vi "cam0config-20GC.vi"(8 "error_in":errorcluster caption="错误输入（无错误）", 10 "Attribute Information Array":T3(array[cluster]), 11 "Session in":T1 caption="Session Out") -> (0 "error_out":errorcluster caption="错误输出", 3 "Session_out":T1)   [LabVIEW 2015]
uses:
  <vilib>/vision/driver/IMAQdx.llb/IMAQdx Attribute Type.ctl
  <vilib>/userdefined/High Color/IMAQdx.ctl
  <resource>/objmgr/imaqdx.rc
  <vilib>/vision/driver/NI_Vision_Acquisition_Software.lvlib
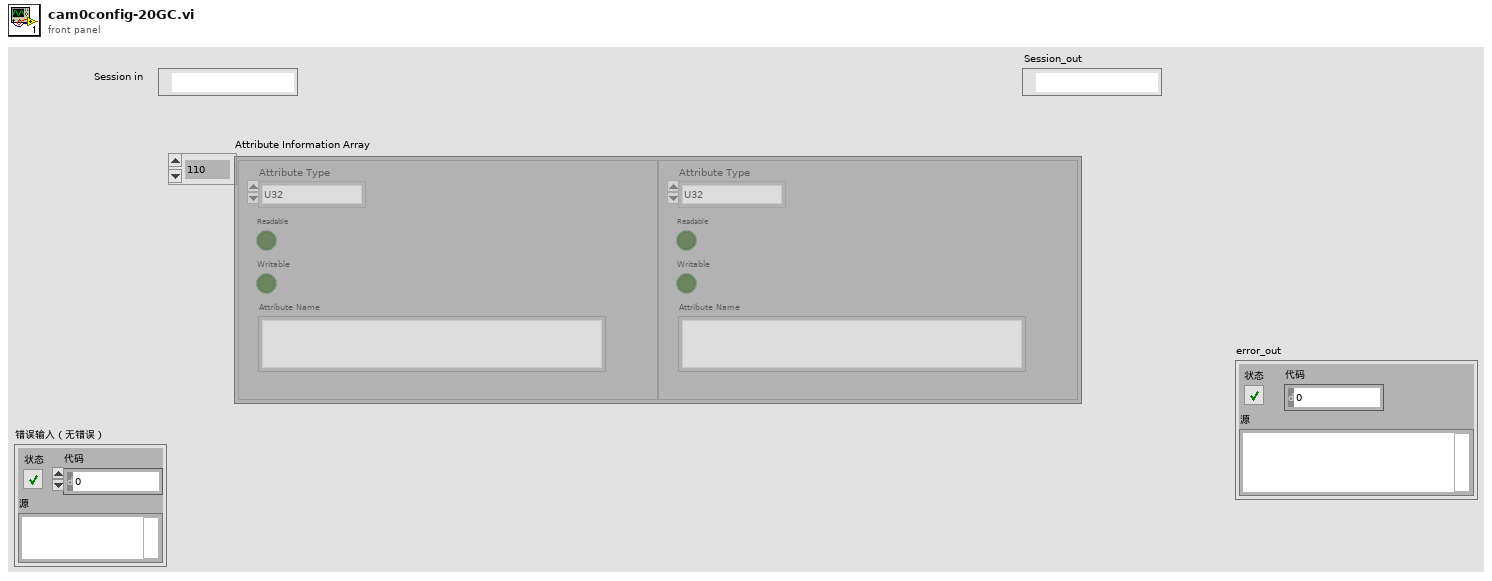
[diagram p1: front panel]
types:
  T1 = typedef "IMAQdx.ctl" = refnum<k21>
  T2 = typedef "NI_Vision_Acquisition_Software.lvlib/IMAQdx Attribute Type.ctl" = enum32{"U32", "I64", "DBL", "String", "Enum", "Bool", "Command"}
  T3 = cluster{"Attribute Type":T2, "Readable":bool, "Writable":bool, "Attribute Name":string}[]
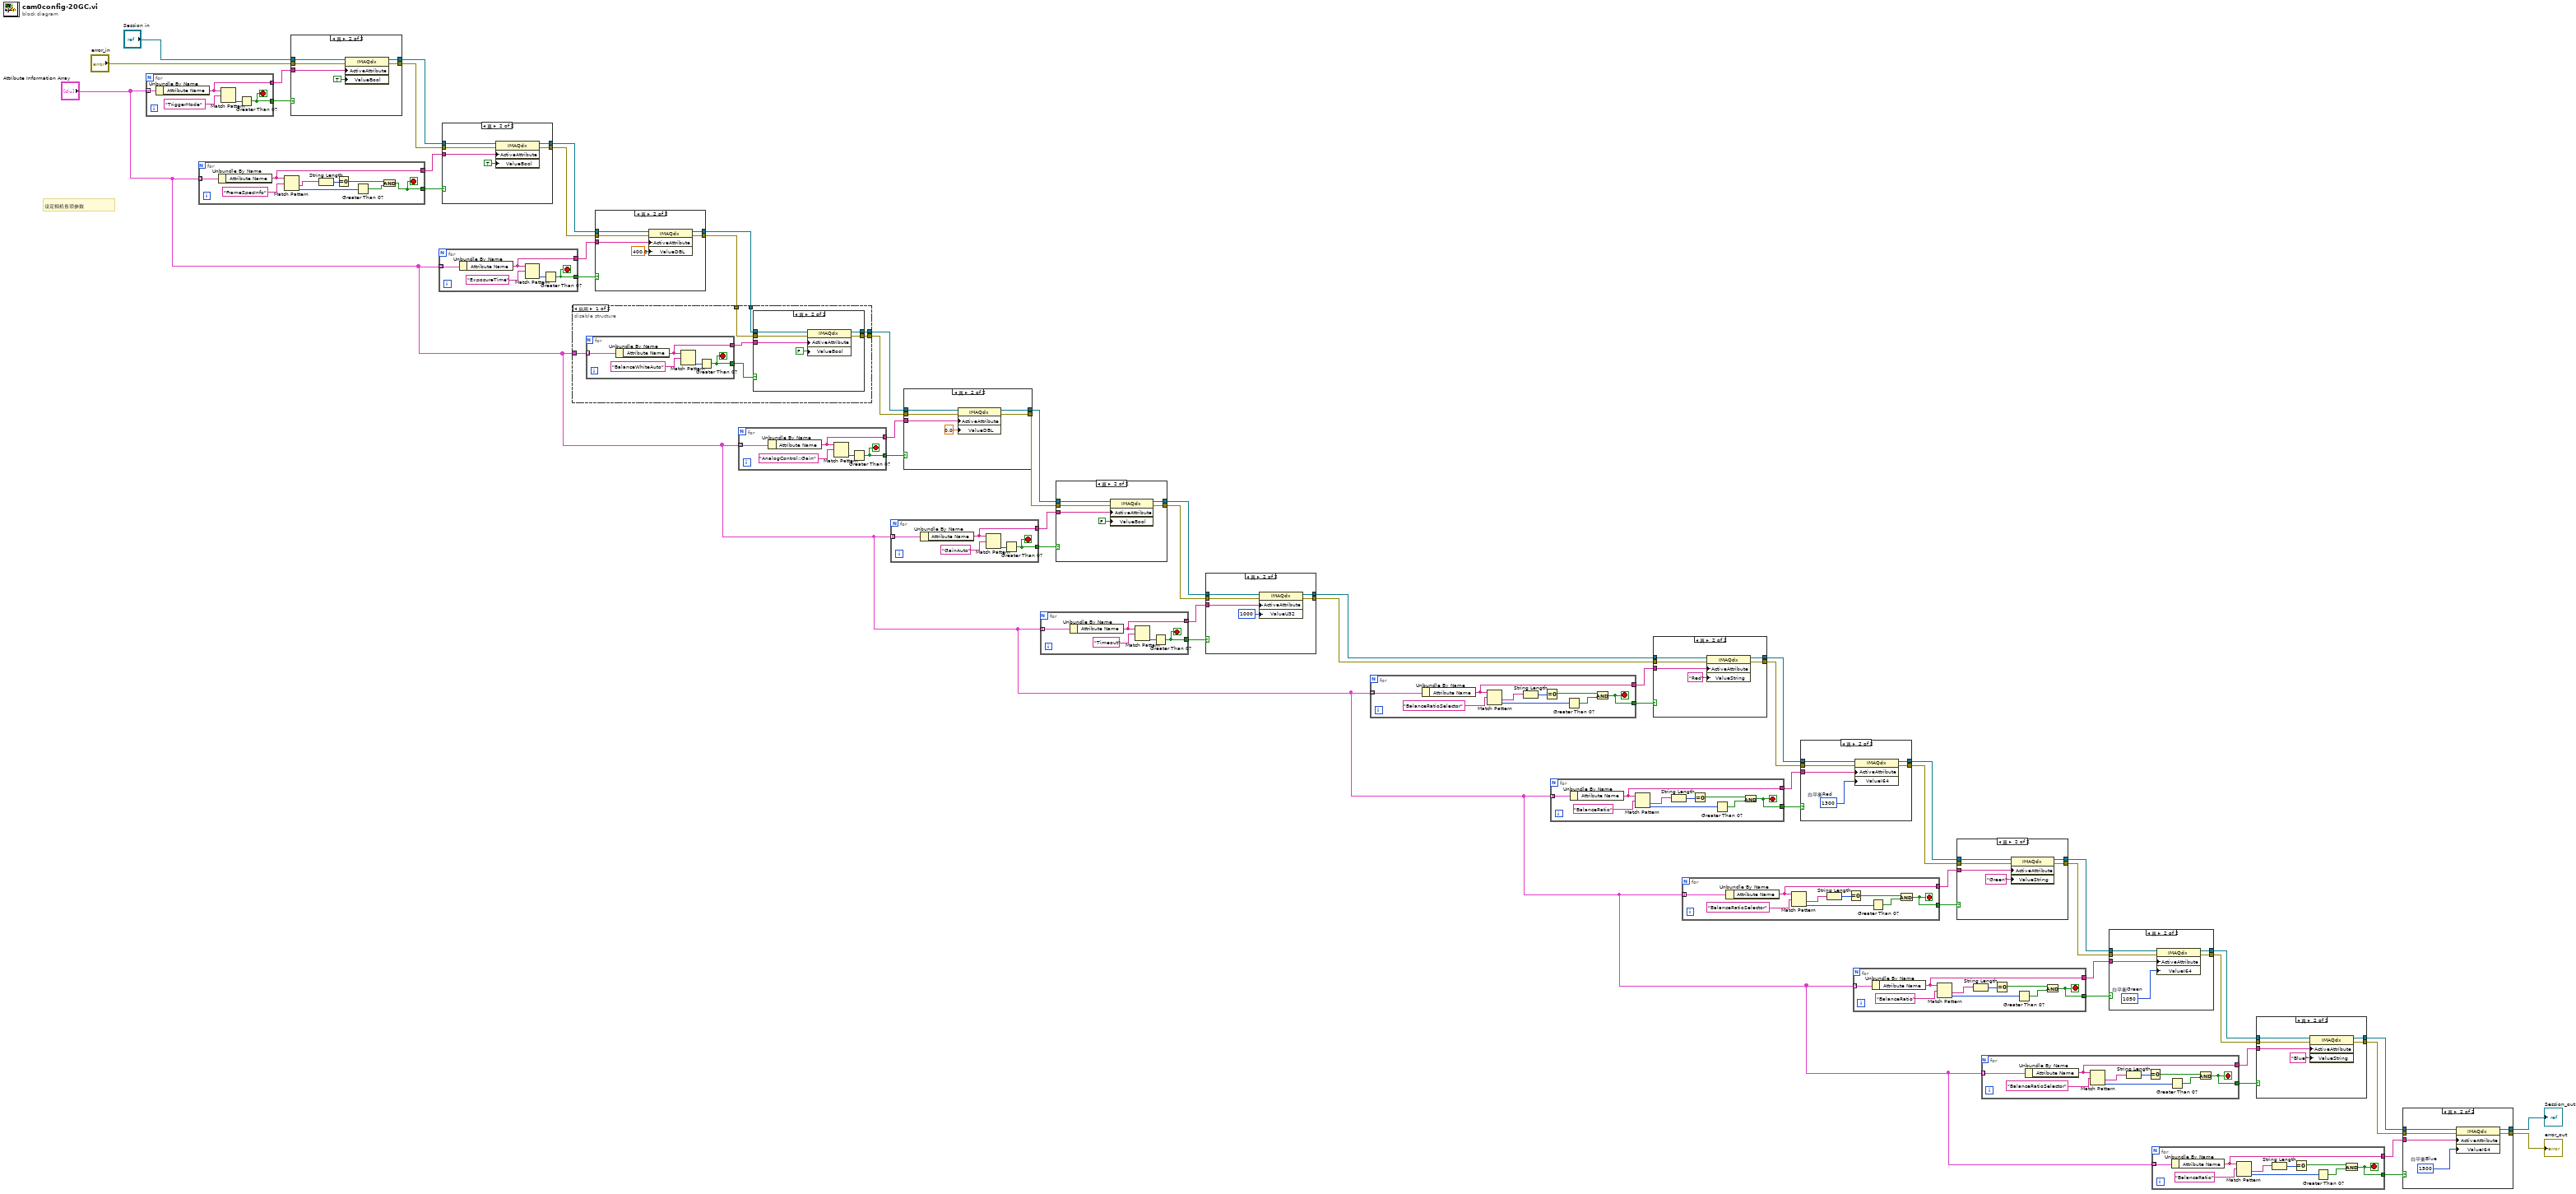
[diagram p0: block diagram]
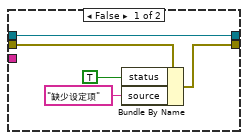
[diagram p2: hidden frame]
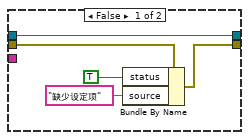
[diagram p3: hidden frame]
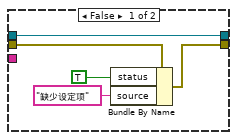
[diagram p4: hidden frame]
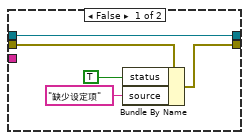
[diagram p5: hidden frame]
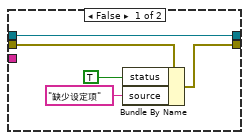
[diagram p6: hidden frame]
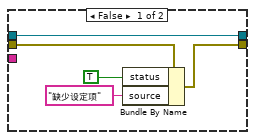
[diagram p7: hidden frame]
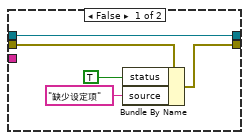
[diagram p8: hidden frame]
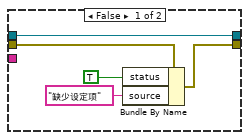
[diagram p10: hidden frame]
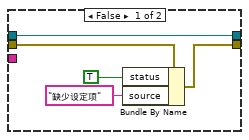
[diagram p11: hidden frame]
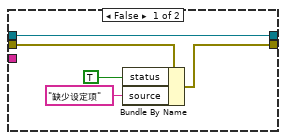
[diagram p12: hidden frame]
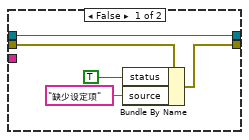
[diagram p13: hidden frame]
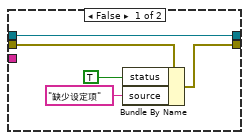
[diagram p14: hidden frame]
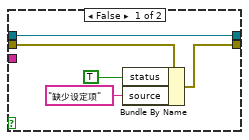
[diagram p15: hidden frame]
diagram:
  # "设定相机各项参数"
  n1 = for {
    tunnel: "Attribute Information Array" -> [w57] mode=indexing
    tunnel: [w55] -> w53
    tunnel: [w54] -> w52
    stop <- w55 stop-if-true
    n2 = Unbundle By Name(w57) -> ("Attribute Name"=w54:string)
    n3 = Match Pattern(string=w54, regular expression="TriggerMode" ("输入字符串")) -> (offset past match=w56:i32)  [unwired: 1 in, 3 out]
    n4 = Greater Than 0?(x=w56) -> (x > 0?=w55:bool)
  }
  n5 = for {
    tunnel: "Attribute Information Array" -> [w66] mode=indexing
    tunnel: [w60] -> w50
    tunnel: [w64] -> w51
    stop <- w60 stop-if-true
    n6 = Unbundle By Name(w66) -> ("Attribute Name"=w64:string)
    n7 = Match Pattern(string=w64, regular expression="FrameSpecInfo" ("输入字符串")) -> (after substring=w63:string, offset past match=w65:i32)  [unwired: 1 in, 2 out]
    n8 = String Length(string=w63) -> (length=w62:i32)
    n9 = Equal To 0?(x=w62) -> (x = 0?=w59:bool)
    n10 = Greater Than 0?(x=w65) -> (x > 0?=w61:bool)
    n11 = And(x=w59, y=w61) -> (x .and. y?=w60:bool)
  }
  n12 = case shown="真" w53 {
    tunnel: "Session in" -> [w72 w78]
    tunnel: w52 -> [_ w77]
    tunnel: [w72 w75] -> w49
    tunnel: "error_in" -> [w71 w74]
    tunnel: [w70 w73] -> w48
    frame False {
      n13 = Bundle By Name(cluster=w71, "status"=TRUE, "source"="缺少设定项") -> (w70:errorcluster)
    }
    frame True {
      n14 = property class="IMAQdx"(reference=w78, error in=w74, "ActiveAttribute"=w77, "ValueBool"=TRUE) -> (reference out=w75:T1, error out=w73:errorcluster)
    }
  }
  n15 = for {
    tunnel: "Attribute Information Array" -> [w82] mode=indexing
    tunnel: [w80] -> w47
    tunnel: [w79] -> w46
    stop <- w80 stop-if-true
    n16 = Unbundle By Name(w82) -> ("Attribute Name"=w79:string)
    n17 = Match Pattern(string=w79, regular expression="ExposureTime" ("输入字符串")) -> (offset past match=w81:i32)  [unwired: 1 in, 3 out]
    n18 = Greater Than 0?(x=w81) -> (x > 0?=w80:bool)
  }
  n19 = case shown="真" w50 {
    tunnel: w49 -> [w88 w94]
    tunnel: w51 -> [_ w93]
    tunnel: [w88 w91] -> w45
    tunnel: w48 -> [w87 w90]
    tunnel: [w86 w89] -> w44
    frame False {
      n20 = Bundle By Name(cluster=w87, "status"=TRUE, "source"="缺少设定项") -> (w86:errorcluster)
    }
    frame True {
      n21 = property class="IMAQdx"(reference=w94, error in=w90, "ActiveAttribute"=w93, "ValueBool"=TRUE) -> (reference out=w91:T1, error out=w89:errorcluster)
    }
  }
  n22 = case shown="真" w47 {
    tunnel: w45 -> [w99 w105]
    tunnel: w46 -> [_ w104]
    tunnel: [w99 w103] -> w43
    tunnel: w44 -> [w98 w102]
    tunnel: [w97 w101] -> w42
    frame False {
      n23 = Bundle By Name(cluster=w98, "status"=TRUE, "source"="缺少设定项") -> (w97:errorcluster)
    }
    frame True {
      n24 = property class="IMAQdx"(reference=w105, error in=w102, "ActiveAttribute"=w104, "ValueDBL"=400.0) -> (reference out=w103:T1, error out=w101:errorcluster)
    }
  }
  n25 = disable-structure shown="启用" {
    disable-tunnel: w43 -> [w110 w129]
    disable-tunnel: w42 -> [w109 w130]
    disable-tunnel: [w108 w129] -> w37
    disable-tunnel: [w107 w130] -> w36
    disable-tunnel: "Attribute Information Array" -> [w106 _]
    frame Enabled {
      n26 = for {
        tunnel: w106 -> [w127] mode=indexing
        tunnel: [w125] -> w111
        tunnel: [w124] -> w112
        stop <- w125 stop-if-true
        n27 = Unbundle By Name(w127) -> ("Attribute Name"=w124:string)
        n28 = Match Pattern(string=w124, regular expression="BalanceWhiteAuto" ("输入字符串")) -> (offset past match=w126:i32)  [unwired: 1 in, 3 out]
        n29 = Greater Than 0?(x=w126) -> (x > 0?=w125:bool)
      }
      n30 = case shown="真" w111 {
        tunnel: w110 -> [w117 w123]
        tunnel: w112 -> [_ w122]
        tunnel: [w117 w121] -> w108
        tunnel: w109 -> [w116 w120]
        tunnel: [w115 w119] -> w107
        frame False {
          n31 = Bundle By Name(cluster=w116, "status"=TRUE, "source"="缺少设定项") -> (w115:errorcluster)
        }
        frame True {
          n32 = property class="IMAQdx"(reference=w123, error in=w120, "ActiveAttribute"=w122, "ValueBool"=FALSE) -> (reference out=w121:T1, error out=w119:errorcluster)
        }
      }
    }
    frame Disabled {
    }
  }
  n33 = for {
    tunnel: "Attribute Information Array" -> [w134] mode=indexing
    tunnel: [w132] -> w41
    tunnel: [w131] -> w40
    stop <- w132 stop-if-true
    n34 = Unbundle By Name(w134) -> ("Attribute Name"=w131:string)
    n35 = Match Pattern(string=w131, regular expression="AnalogControl::Gain" ("输入字符串")) -> (offset past match=w133:i32)  [unwired: 1 in, 3 out]
    n36 = Greater Than 0?(x=w133) -> (x > 0?=w132:bool)
  }
  n37 = for {
    tunnel: "Attribute Information Array" -> [w139] mode=indexing
    tunnel: [w137] -> w38
    tunnel: [w136] -> w39
    stop <- w137 stop-if-true
    n38 = Unbundle By Name(w139) -> ("Attribute Name"=w136:string)
    n39 = Match Pattern(string=w136, regular expression="GainAuto" ("输入字符串")) -> (offset past match=w138:i32)  [unwired: 1 in, 3 out]
    n40 = Greater Than 0?(x=w138) -> (x > 0?=w137:bool)
  }
  n41 = case shown="真" w41 {
    tunnel: w37 -> [w145 w151]
    tunnel: w40 -> [_ w150]
    tunnel: [w145 w149] -> w35
    tunnel: w36 -> [w144 w148]
    tunnel: [w143 w147] -> w34
    frame False {
      n42 = Bundle By Name(cluster=w144, "status"=TRUE, "source"="缺少设定项") -> (w143:errorcluster)
    }
    frame True {
      n43 = property class="IMAQdx"(reference=w151, error in=w148, "ActiveAttribute"=w150, "ValueDBL"=0.0) -> (reference out=w149:T1, error out=w147:errorcluster)
    }
  }
  n44 = for {
    tunnel: "Attribute Information Array" -> [w155] mode=indexing
    tunnel: [w153] -> w31
    tunnel: [w152] -> w30
    stop <- w153 stop-if-true
    n45 = Unbundle By Name(w155) -> ("Attribute Name"=w152:string)
    n46 = Match Pattern(string=w152, regular expression="Timeout" ("输入字符串")) -> (offset past match=w154:i32)  [unwired: 1 in, 3 out]
    n47 = Greater Than 0?(x=w154) -> (x > 0?=w153:bool)
  }
  n48 = case shown="真" w38 {
    tunnel: w35 -> [w161 w167]
    tunnel: w39 -> [_ w166]
    tunnel: [w161 w165] -> w29
    tunnel: w34 -> [w160 w164]
    tunnel: [w159 w163] -> w28
    frame False {
      n49 = Bundle By Name(cluster=w160, "status"=TRUE, "source"="缺少设定项") -> (w159:errorcluster)
    }
    frame True {
      n50 = property class="IMAQdx"(reference=w167, error in=w164, "ActiveAttribute"=w166, "ValueBool"=FALSE) -> (reference out=w165:T1, error out=w163:errorcluster)
    }
  }
  n51 = case shown="真" w31 {
    tunnel: w29 -> [w172 w178]
    tunnel: w30 -> [_ w177]
    tunnel: [w172 w176] -> w3
    tunnel: w28 -> [w171 w175]
    tunnel: [w170 w174] -> w2
    frame False {
      n52 = Bundle By Name(cluster=w171, "status"=TRUE, "source"="缺少设定项") -> (w170:errorcluster)
    }
    frame True {
      n53 = property class="IMAQdx"(reference=w178, error in=w175, "ActiveAttribute"=w177, "ValueU32"=u32 1000) -> (reference out=w176:T1, error out=w174:errorcluster)
    }
  }
  n54 = for {
    tunnel: "Attribute Information Array" -> [w187] mode=indexing
    tunnel: [w180] -> w26
    tunnel: [w185] -> w27
    stop <- w180 stop-if-true
    n55 = Unbundle By Name(w187) -> ("Attribute Name"=w185:string)
    n56 = Match Pattern(string=w185, regular expression="BalanceRatioSelector" ("输入字符串")) -> (after substring=w183:string, offset past match=w186:i32)  [unwired: 1 in, 2 out]
    n57 = String Length(string=w183) -> (length=w184:i32)
    n58 = Equal To 0?(x=w184) -> (x = 0?=w182:bool)
    n59 = Greater Than 0?(x=w186) -> (x > 0?=w181:bool)
    n60 = And(x=w182, y=w181) -> (x .and. y?=w180:bool)
  }
  n61 = for {
    tunnel: "Attribute Information Array" -> [w196] mode=indexing
    tunnel: [w189] -> w25
    tunnel: [w194] -> w24
    stop <- w189 stop-if-true
    n62 = Unbundle By Name(w196) -> ("Attribute Name"=w194:string)
    n63 = Match Pattern(string=w194, regular expression="BalanceRatio" ("输入字符串")) -> (after substring=w192:string, offset past match=w195:i32)  [unwired: 1 in, 2 out]
    n64 = String Length(string=w192) -> (length=w193:i32)
    n65 = Equal To 0?(x=w193) -> (x = 0?=w191:bool)
    n66 = Greater Than 0?(x=w195) -> (x > 0?=w190:bool)
    n67 = And(x=w191, y=w190) -> (x .and. y?=w189:bool)
  }
  n68 = case shown="真" w26 {
    tunnel: w3 -> [w201 w207]
    tunnel: w27 -> [_ w206]
    tunnel: [w201 w205] -> w20
    tunnel: w2 -> [w200 w204]
    tunnel: [w199 w203] -> w21
    frame False {
      n69 = Bundle By Name(cluster=w200, "status"=TRUE, "source"="缺少设定项") -> (w199:errorcluster)
    }
    frame True {
      n70 = property class="IMAQdx"(reference=w207, error in=w204, "ActiveAttribute"=w206, "ValueString"="Red") -> (reference out=w205:T1, error out=w203:errorcluster)
    }
  }
  n71 = for {
    tunnel: "Attribute Information Array" -> [w216] mode=indexing
    tunnel: [w209] -> w22
    tunnel: [w214] -> w23
    stop <- w209 stop-if-true
    n72 = Unbundle By Name(w216) -> ("Attribute Name"=w214:string)
    n73 = Match Pattern(string=w214, regular expression="BalanceRatioSelector" ("输入字符串")) -> (after substring=w212:string, offset past match=w215:i32)  [unwired: 1 in, 2 out]
    n74 = String Length(string=w212) -> (length=w213:i32)
    n75 = Equal To 0?(x=w213) -> (x = 0?=w211:bool)
    n76 = Greater Than 0?(x=w215) -> (x > 0?=w210:bool)
    n77 = And(x=w211, y=w210) -> (x .and. y?=w209:bool)
  }
  n78 = case shown="真" w25 {
    tunnel: w20 -> [w221 w227]
    tunnel: w24 -> [_ w226]
    tunnel: [w221 w225] -> w18
    tunnel: w21 -> [w220 w224]
    tunnel: [w219 w223] -> w19
    frame False {
      n79 = Bundle By Name(cluster=w220, "status"=TRUE, "source"="缺少设定项") -> (w219:errorcluster)
    }
    frame True {
      w222 = i64 1300  # 白平衡Red
      n80 = property class="IMAQdx"(reference=w227, error in=w224, "ActiveAttribute"=w226, "ValueI64"=w222) -> (reference out=w225:T1, error out=w223:errorcluster)
    }
  }
  n81 = for {
    tunnel: "Attribute Information Array" -> [w236] mode=indexing
    tunnel: [w229] -> w16
    tunnel: [w234] -> w17
    stop <- w229 stop-if-true
    n82 = Unbundle By Name(w236) -> ("Attribute Name"=w234:string)
    n83 = Match Pattern(string=w234, regular expression="BalanceRatio" ("输入字符串")) -> (after substring=w232:string, offset past match=w235:i32)  [unwired: 1 in, 2 out]
    n84 = String Length(string=w232) -> (length=w233:i32)
    n85 = Equal To 0?(x=w233) -> (x = 0?=w231:bool)
    n86 = Greater Than 0?(x=w235) -> (x > 0?=w230:bool)
    n87 = And(x=w231, y=w230) -> (x .and. y?=w229:bool)
  }
  n88 = case shown="真" w22 {
    tunnel: w18 -> [w241 w247]
    tunnel: w23 -> [_ w246]
    tunnel: [w241 w245] -> w14
    tunnel: w19 -> [w240 w244]
    tunnel: [w239 w243] -> w15
    frame False {
      n89 = Bundle By Name(cluster=w240, "status"=TRUE, "source"="缺少设定项") -> (w239:errorcluster)
    }
    frame True {
      n90 = property class="IMAQdx"(reference=w247, error in=w244, "ActiveAttribute"=w246, "ValueString"="Green") -> (reference out=w245:T1, error out=w243:errorcluster)
    }
  }
  n91 = for {
    tunnel: "Attribute Information Array" -> [w256] mode=indexing
    tunnel: [w249] -> w9
    tunnel: [w254] -> w8
    stop <- w249 stop-if-true
    n92 = Unbundle By Name(w256) -> ("Attribute Name"=w254:string)
    n93 = Match Pattern(string=w254, regular expression="BalanceRatioSelector" ("输入字符串")) -> (after substring=w252:string, offset past match=w255:i32)  [unwired: 1 in, 2 out]
    n94 = String Length(string=w252) -> (length=w253:i32)
    n95 = Equal To 0?(x=w253) -> (x = 0?=w251:bool)
    n96 = Greater Than 0?(x=w255) -> (x > 0?=w250:bool)
    n97 = And(x=w251, y=w250) -> (x .and. y?=w249:bool)
  }
  n98 = case shown="真" w16 {
    tunnel: w14 -> [w261 w267]
    tunnel: w17 -> [_ w266]
    tunnel: [w261 w265] -> w6
    tunnel: w15 -> [w260 w264]
    tunnel: [w259 w263] -> w7
    frame False {
      n99 = Bundle By Name(cluster=w260, "status"=TRUE, "source"="缺少设定项") -> (w259:errorcluster)
    }
    frame True {
      w262 = i64 1050  # 白平衡Green
      n100 = property class="IMAQdx"(reference=w267, error in=w264, "ActiveAttribute"=w266, "ValueI64"=w262) -> (reference out=w265:T1, error out=w263:errorcluster)
    }
  }
  n101 = for {
    tunnel: "Attribute Information Array" -> [w276] mode=indexing
    tunnel: [w269] -> w11
    tunnel: [w274] -> w10
    stop <- w269 stop-if-true
    n102 = Unbundle By Name(w276) -> ("Attribute Name"=w274:string)
    n103 = Match Pattern(string=w274, regular expression="BalanceRatio" ("输入字符串")) -> (after substring=w272:string, offset past match=w275:i32)  [unwired: 1 in, 2 out]
    n104 = String Length(string=w272) -> (length=w273:i32)
    n105 = Equal To 0?(x=w273) -> (x = 0?=w271:bool)
    n106 = Greater Than 0?(x=w275) -> (x > 0?=w270:bool)
    n107 = And(x=w271, y=w270) -> (x .and. y?=w269:bool)
  }
  n108 = case shown="真" w9 {
    tunnel: w6 -> [w281 w287]
    tunnel: w8 -> [_ w286]
    tunnel: [w281 w285] -> w13
    tunnel: w7 -> [w280 w284]
    tunnel: [w279 w283] -> w12
    frame False {
      n109 = Bundle By Name(cluster=w280, "status"=TRUE, "source"="缺少设定项") -> (w279:errorcluster)
    }
    frame True {
      n110 = property class="IMAQdx"(reference=w287, error in=w284, "ActiveAttribute"=w286, "ValueString"="Blue") -> (reference out=w285:T1, error out=w283:errorcluster)
    }
  }
  n111 = case shown="真" w11 {
    tunnel: w13 -> [w292 w298]
    tunnel: w10 -> [_ w297]
    tunnel: [w292 w296] -> w5
    tunnel: w12 -> [w291 w295]
    tunnel: [w290 w294] -> w4
    frame False {
      n112 = Bundle By Name(cluster=w291, "status"=TRUE, "source"="缺少设定项") -> (w290:errorcluster)
    }
    frame True {
      w293 = i64 1500  # 白平衡Blue
      n113 = property class="IMAQdx"(reference=w298, error in=w295, "ActiveAttribute"=w297, "ValueI64"=w293) -> (reference out=w296:T1, error out=w294:errorcluster)
    }
  }
  "error_out" <- w4
  "Session_out" <- w5
